vi "NIIE_MoveLayers.vi"(8 "Error":errorcluster, 10 "Arrow Up":bool, 11 "Data":T1={"Class"={"Ants"=refnum, "Layer"=refnum, "Templates"=refnum, "Icon"=refnum, "Glyph"=refnum, "Settings"=refnum, "Tools"=refnum}, "Ref"={"Add Layer"=refnum, "Remove Layer"=refnum, "Line Text"=[], "Body Text Spec"=refnum, "DNL_Font"=refnum, "glyph path str"=refnum, "templates path str"=refnum, "Arrow Up"=refnum, "Arrow Down"=refnum, "IE VI Ref"=refnum, "Glyphs tree"=refnum, "Templates tree"=refnum, "Layer Icon Text"=refnum, "Layer Template"=refnum, "Clipboard"=refnum, "BW icon in"=refnum, "Color icon in"=refnum, "Layer Clust"=refnum, "Body Text"=refnum, "DNL_Framework Templates"=refnum, "Search Templates"=refnum, "TextMarker"=refnum, "Tab Control"=refnum, "Search Glyphs"=refnum, "Line Color"=refnum, "DNL_Glyphs []"=refnum, "Fill Color"=refnum, "Tools"=refnum, "Glyphs tree"=refnum, "Icon"=refnum, "Preview"=refnum, "Ants"=refnum, "Terminals"=refnum, "menu reference"=refnum, "LayerNames"=[], "GlyphLoadAnimation"=refnum, "TemplateLoadAnimation"=refnum, "refreshGlyphs"=refnum, "refreshTemplates"=refnum}, "Support"={"AntsRect"={"left"=0, "top"=0, "right"=0, "bottom"=0}, "Mouse Move Coords"={"Horizontal"=0, "Vertical"=0}, "Mouse Down Coords"={"Horizontal"=0, "Vertical"=0}, "Temp Coord"={"Horizontal"=0, "Vertical"=0}, "Action"=enum."Default", "Edge Color"=4914962, "Fill Color"=16860, "Mouse Down?"=FALSE, "Draft Mode?"=FALSE, "Temp Icon"=bytes[3102], "CTRL Pressed"=FALSE, "Move Selection?"=FALSE, "AntsRect Orig"={"left"=0, "top"=0, "right"=0, "bottom"=0}, "Text"="", "TM Set?"=FALSE, "Mouse inside icon?"=FALSE, "Tool (old value)"=0, "Pencil Move Color"=0, "Swap Colors?"=FALSE, "Shift pressed?"=FALSE}}) -> (0 "Error Out":errorcluster, 3 "Data Out":T1={"Class"={"Ants"=refnum, "Layer"=refnum, "Templates"=refnum, "Icon"=refnum, "Glyph"=refnum, "Settings"=refnum, "Tools"=refnum}, "Ref"={"Add Layer"=refnum, "Remove Layer"=refnum, "Line Text"=[], "Body Text Spec"=refnum, "DNL_Font"=refnum, "glyph path str"=refnum, "templates path str"=refnum, "Arrow Up"=refnum, "Arrow Down"=refnum, "IE VI Ref"=refnum, "Glyphs tree"=refnum, "Templates tree"=refnum, "Layer Icon Text"=refnum, "Layer Template"=refnum, "Clipboard"=refnum, "BW icon in"=refnum, "Color icon in"=refnum, "Layer Clust"=refnum, "Body Text"=refnum, "DNL_Framework Templates"=refnum, "Search Templates"=refnum, "TextMarker"=refnum, "Tab Control"=refnum, "Search Glyphs"=refnum, "Line Color"=refnum, "DNL_Glyphs []"=refnum, "Fill Color"=refnum, "Tools"=refnum, "Glyphs tree"=refnum, "Icon"=refnum, "Preview"=refnum, "Ants"=refnum, "Terminals"=refnum, "menu reference"=refnum, "LayerNames"=[], "GlyphLoadAnimation"=refnum, "TemplateLoadAnimation"=refnum, "refreshGlyphs"=refnum, "refreshTemplates"=refnum}, "Support"={"AntsRect"={"left"=0, "top"=0, "right"=0, "bottom"=0}, "Mouse Move Coords"={"Horizontal"=0, "Vertical"=0}, "Mouse Down Coords"={"Horizontal"=0, "Vertical"=0}, "Temp Coord"={"Horizontal"=0, "Vertical"=0}, "Action"=enum."Default", "Edge Color"=4914962, "Fill Color"=16860, "Mouse Down?"=FALSE, "Draft Mode?"=FALSE, "Temp Icon"=bytes[3102], "CTRL Pressed"=FALSE, "Move Selection?"=FALSE, "AntsRect Orig"={"left"=0, "top"=0, "right"=0, "bottom"=0}, "Text"="", "TM Set?"=FALSE, "Mouse inside icon?"=FALSE, "Tool (old value)"=0, "Pencil Move Color"=0, "Swap Colors?"=FALSE, "Shift pressed?"=FALSE}})   [LabVIEW 2021]
uses:
  Controls/IE Data.ctl
  Class/Ants/Ants.lvclass
  Class/FakedArray/FakedArray.lvclass
  Class/Icon Library/Glyph.lvclass
  Class/Settings/Settings.lvclass
  Class/Tools/Tools Paint.lvclass
  vi.lib/LabVIEW Icon API/lv_icon/Classes/Icon/Icon.lvclass
  Controls/IE Classes.ctl
  Controls/References Cluster.ctl
  Controls/SupportClass.ctl
  <vilib>/Utility/miscctls.llb/LVPoint32TypeDef.ctl
  Controls/ENUM_SupportClass_Action.ctl
  vi.lib/LabVIEW Icon API/lv_icon/Controls/IEColor.ctl
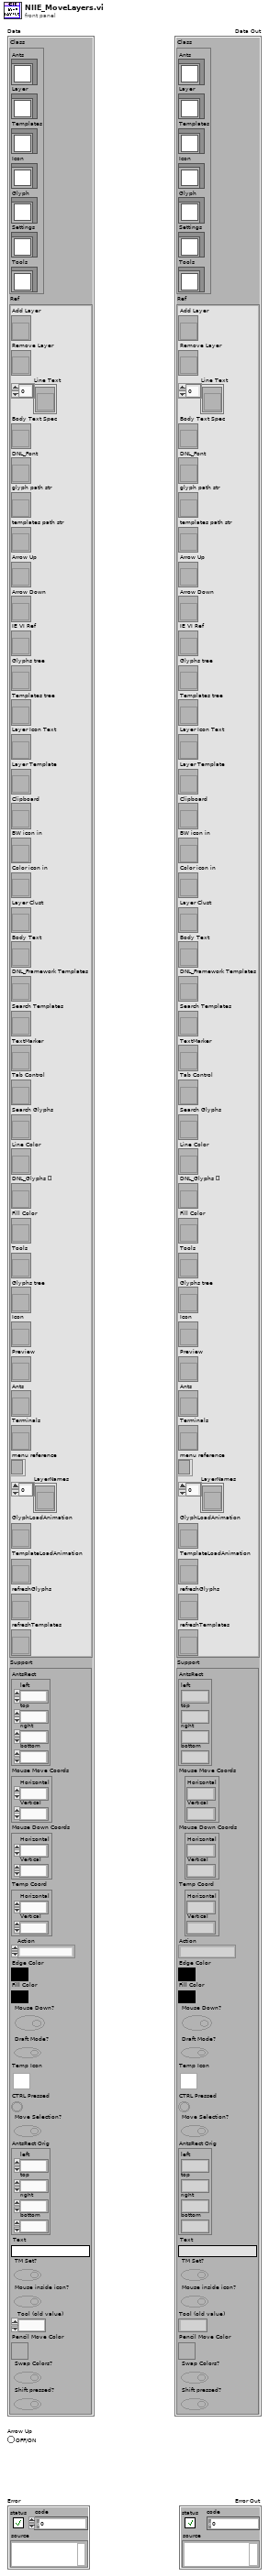
[diagram p1: front panel]
types:
  T1 = typedef "IE Data.ctl" = cluster{"Class":T2, "Ref":T3, "Support":T4}
  T2 = typedef "IE Classes.ctl" = cluster{"Ants":refnum<class "Ants.lvclass">, "Layer":refnum<class "FakedArray.lvclass">, "Templates":refnum<class "FakedArray.lvclass">, "Icon":refnum<class "Icon.lvclass">, "Glyph":refnum<class "Glyph.lvclass">, "Settings":refnum<class "Settings.lvclass">, "Tools":refnum<class "Tools Paint.lvclass">}
  T3 = typedef "References Cluster.ctl" = cluster{"Add Layer":refnum<vi>, "Remove Layer":refnum<vi>, "Line Text":refnum<vi>[], "Body Text Spec":refnum<vi>, "DNL_Font":refnum<vi>, "glyph path str":refnum<vi>, "templates path str":refnum<vi>, "Arrow Up":refnum<vi>, "Arrow Down":refnum<vi>, "IE VI Ref":refnum<vi>, "Glyphs tree":refnum<vi>, "Templates tree":refnum<vi>, "Layer Icon Text":refnum<vi>, "Layer Template":refnum<vi>, "Clipboard":refnum<vi>, "BW icon in":refnum<vi>, "Color icon in":refnum<vi>, "Layer Clust":refnum<vi>, "Body Text":refnum<vi>, "DNL_Framework Templates":refnum<vi>, "Search Templates":refnum<vi>, "TextMarker":refnum<vi>, "Tab Control":refnum<vi>, "Search Glyphs":refnum<vi>, "Line Color":refnum<vi>, "DNL_Glyphs []":refnum<vi>, "Fill Color":refnum<vi>, "Tools":refnum<vi>, "Glyphs tree":refnum<vi>, "Icon":refnum<vi>, "Preview":refnum<vi>, "Ants":refnum<vi>, "Terminals":refnum<vi>, "menu reference":refnum<k9>, "LayerNames":refnum<vi>[], "GlyphLoadAnimation":refnum<vi>, "TemplateLoadAnimation":refnum<vi>, "refreshGlyphs":refnum<vi>, "refreshTemplates":refnum<vi>}
  T4 = typedef "SupportClass.ctl" = cluster{"AntsRect":cluster{"left":i16, "top":i16, "right":i16, "bottom":i16}, "Mouse Move Coords":T5, "Mouse Down Coords":T5, "Temp Coord":T5, "Action":T6, "Edge Color":T7, "Fill Color":T7, "Mouse Down?":bool, "Draft Mode?":bool, "Temp Icon":picture, "CTRL Pressed":bool, "Move Selection?":bool, "AntsRect Orig":cluster{"left":i16, "top":i16, "right":i16, "bottom":i16}, "Text":string, "TM Set?":bool, "Mouse inside icon?":bool, "Tool (old value)":u32, "Pencil Move Color":u32, "Swap Colors?":bool, "Shift pressed?":bool}
  T5 = typedef "LVPoint32TypeDef.ctl" = cluster{"Horizontal":i32, "Vertical":i32}
  T6 = typedef "ENUM_SupportClass_Action.ctl" = enum16{"Default", "Move Selection", "Glyph Library", "Tool"}
  T7 = typedef "IEColor.ctl" = u32
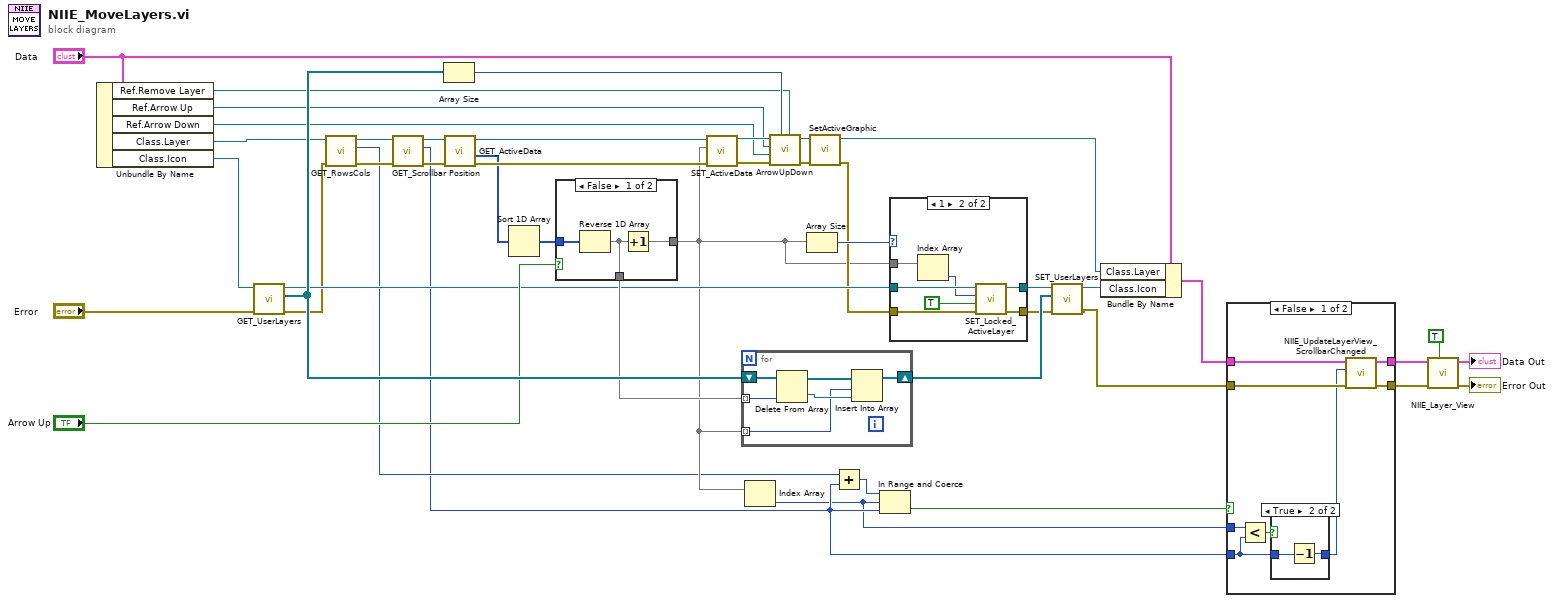
[diagram p0: block diagram]
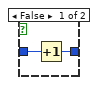
[diagram p2: hidden frame]
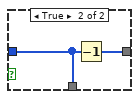
[diagram p5: hidden frame]
diagram:
  n1 = Unbundle By Name("Data") -> ("Ref.Remove Layer"=w1:refnum<vi>, "Ref.Arrow Up"=w20:refnum<vi>, "Ref.Arrow Down"=w21:refnum<vi>, "Class.Layer"=w6:refnum<class "FakedArray.lvclass">, "Class.Icon"=w25:refnum<class "Icon.lvclass">)
  n2 = call-dynamic "GET_UserLayers.vi"("error in (no error)"="Error", "Icon.lvclass in"=w25) -> ("error out"=w9:errorcluster, "All Layers"=w39:refnum<class "Layer.lvclass">[], "Icon.lvclass out"=w27:refnum<class "Icon.lvclass">)  [unwired: 7 out]
  n3 = call-dynamic "GET_RowsCols.vi"("error in (no error)"=w9, "FakedArray.lvclass in"=w6) -> ("error out"=w8:errorcluster, "# Rows"=w5:i32, "FakedArray.lvclass out"=w7:refnum<class "FakedArray.lvclass">)  [unwired: 7 out]
  n4 = call-dynamic "GET_Scrollbar Position.vi"("error in (no error)"=w8, "FakedArray.lvclass in"=w7) -> ("error out"=w10:errorcluster, "Scrollbar Position"=w3:i32, "FakedArray.lvclass out"=w11:refnum<class "FakedArray.lvclass">)  [unwired: 7 out]
  n5 = Array Size(array=w39) -> (size(s)=w38:i32)
  n6 = call-dynamic "GET_ActiveData.vi"("Error"=w10, "FakedArray"=w11) -> ("Error Out"=w45:errorcluster, "Active Data [] Out"=w34:i32[], "FakedArray Out"=w41:refnum<class "FakedArray.lvclass">)  [unwired: 7 out]
  n7 = Sort 1D Array(array=w34) -> (sorted array=w32:i32[])
  n8 = case shown="False" "Arrow Up" {
    tunnel: w32 -> [w48 w49]
    tunnel: [w47 w50] -> w12
    tunnel: [w46 w49] -> w31
    frame False {
      n9 = Reverse 1D Array(array=w48) -> (reversed array=w46:i32[])
      n10 = Increment(x=w46) -> (x+1=w47:i32[])
    }
    frame True {
      n11 = Decrement(x=w49) -> (x-1=w50:i32[])
    }
  }
  n12 = call-dynamic "SET_ActiveData.vi"("error in (no error)"=w45, "Active Data"=w12, "FakedArray.lvclass in"=w41) -> ("error out"=w42:errorcluster, "FakedArray.lvclass out"=w40:refnum<class "FakedArray.lvclass">)  [unwired: 7 out]
  n13 = for {
    shift-right: [w53] -> w44
    shift-left: w39 -> [w56]
    tunnel: w31 -> [w55] mode=indexing
    tunnel: w12 -> [w51] mode=indexing
    n14 = Delete From Array(array=w56, index=w55) -> (deleted portion=w52:refnum<class "Layer.lvclass">, array with subset deleted=w54:refnum<class "Layer.lvclass">[])  [unwired: 1 in]
    n15 = Insert Into Array(array=w54, index=w51, new element=w52) -> (w53:refnum<class "Layer.lvclass">[])
  }
  n16 = Index Array(array=w12) -> (element=w2:i32)  [unwired: 1 in]
  n17 = call "ArrowUpDown.vi"("Remove Layer"=w1, "# Layers"=w38, "Error"=w42, "Arrow Down"=w21, "Arrow Up"=w20, "FakedArray"=w40) -> ("Error Out"=w35:errorcluster, "FakedArray Out"=w36:refnum<class "FakedArray.lvclass">)  [unwired: 4 out]
  n18 = Array Size(array=w12) -> (size(s)=w28:i32)
  n19 = call-dynamic "SetActiveGraphic.vi"("error in (no error)"=w35, "FakedArray in"=w36) -> ("error out"=w26:errorcluster, "FakedArray out"=w19:refnum<class "FakedArray.lvclass">)  [unwired: 4 in, 4 out]
  n20 = Add(x=w5, y=w3) -> (x+y=w13:i32)
  n21 = In Range and Coerce(upper limit=w13, x=w2, lower limit=w3) -> (In Range?=w4:bool)  [unwired: 1 out]
  n22 = case shown="1" w28 {
    tunnel: [w58 w65] -> w30
    tunnel: [w57 w64] -> w29
    tunnel: w27 -> [w58 w63]
    tunnel: w26 -> [w57 w62]
    tunnel: w12 -> [_ w61]
    frame 0, Default {
    }
    frame 1 {
      n23 = Index Array(array=w61) -> (element=w60:i32)  [unwired: 1 in]
      n24 = call-dynamic "SET_Locked_ActiveLayer.vi"("error in (no error)"=w62, "Layers Locked?"=TRUE, "Active Layer"=w60, "Icon.lvclass in"=w63) -> ("error out"=w64:errorcluster, "Icon.lvclass out"=w65:refnum<class "Icon.lvclass">)  [unwired: 6 out]
    }
  }
  n25 = call-dynamic "SET_UserLayers.vi"("error in (no error)"=w29, "Layers"=w44, "Icon.lvclass in"=w30) -> ("error out"=w15:errorcluster, "Icon.lvclass out"=w23:refnum<class "Icon.lvclass">)  [unwired: 7 in]
  n26 = Bundle By Name(cluster="Data", "Class.Layer"=w19, "Class.Icon"=w23) -> (w16:T1)
  n27 = case shown="False" w4 {
    tunnel: [w73 w79] -> w17
    tunnel: w16 -> [w72 w79]
    tunnel: w15 -> [w71 w78]
    tunnel: [w70 w78] -> w14
    tunnel: w3 -> [w66 _]
    tunnel: w2 -> [w67 _]
    frame False {
      n28 = Less?(x=w67, y=w66) -> (x < y?=w69:bool)
      n29 = case shown="True" w69 {
        tunnel: w66 -> [w75 w77]
        tunnel: [w74 w76] -> w68
        frame False {
          n30 = Increment(x=w75) -> (x+1=w74:i32)
        }
        frame True {
          n31 = Decrement(x=w77) -> (x-1=w76:i32)
        }
      }
      n32 = call "NIIE_UpdateLayerView_ScrollbarChanged.vi"("Error"=w71, "Scrollbar Position"=w68, "Data"=w72) -> ("Error Out"=w70:errorcluster, "Data Out"=w73:T1)  [unwired: 7 out]
    }
    frame True {
    }
  }
  n33 = call "NIIE_Layer_View.vi"("Add To Undo?"=TRUE ("Add to Undo?"), "Error"=w14, "Data"=w17) -> ("Error Out"=→"Error Out":errorcluster, "Data Out"=→"Data Out":T1)  [unwired: 2 in, 5 out]
